vi "check_expand_needed.vi"(8 "error in (no error)":errorcluster, 9 "Insert Pos":dbl, 10 "Insert Image":T1, 11 "Larger Image":T1) -> (0 "error out":errorcluster, 1 "Right":bool, 2 "Left":bool, 3 "Either":bool)   [LabVIEW 2016]
doc: "Checks if a horizontal image line added to a larger image, centred at x position 'insert pos', \nwill extend beyond the boundaries of the larger image. Returns true if outside image."
uses:
  <vilib>/vision/Image Controls.llb/IMAQ Image.ctl
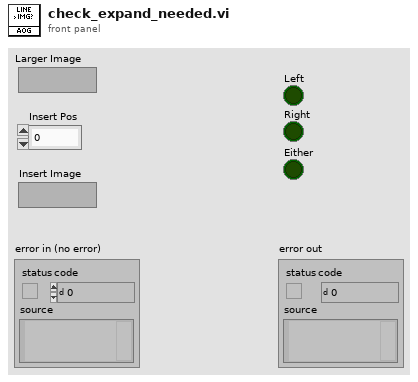
[diagram p1: front panel]
types:
  T1 = typedef "IMAQ Image.ctl" = refnum<image>
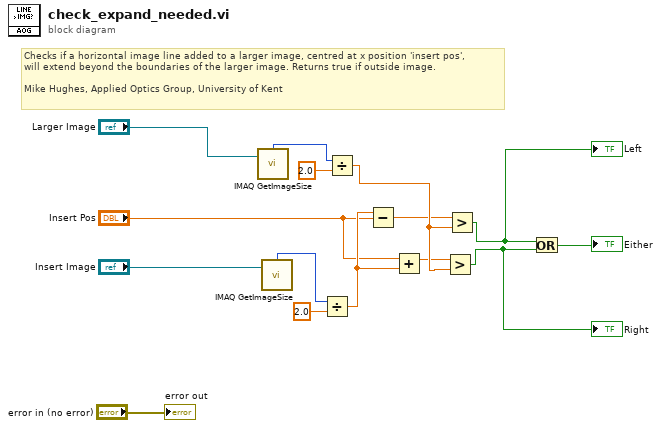
[diagram p0: block diagram]
diagram:
  # "Checks if a horizontal image line added to a larger image, centred at x position 'insert pos', \nwill extend beyond the boundaries of the larger image. Returns true if outside image.\n\nMike Hughes, Applied Optics Group, University of Kent"
  n1 = call "IMAQ GetImageSize"("Image"="Larger Image") -> ("X Resolution"=w15:i32)  [unwired: 3 in, 2 out]
  n2 = call "IMAQ GetImageSize"("Image"="Insert Image") -> ("X Resolution"=w7:i32)  [unwired: 3 in, 2 out]
  n3 = Divide(x=w7, y=2.0) -> (x/y=w12:dbl)
  n4 = Divide(x=w15, y=2.0) -> (x/y=w13:dbl)
  n5 = Subtract(x=w12, y="Insert Pos") -> (x-y=w11:dbl)
  n6 = Add(x="Insert Pos", y=w12) -> (x+y=w10:dbl)
  n7 = Greater?(x=w10, y=w13) -> (0:w3:bool)
  "Right" <- w3
  n8 = Greater?(x=w11, y=w13) -> (0:w14:bool)
  "Left" <- w14
  n9 = Or(x=w14, y=w3) -> (x .or. y?=→"Either":bool)
  "error out" <- "error in (no error)"
